vi "Find Relative Goal Location.vi"(10 "Goal Position":dbl[](array[numeric]), 11 "Current Position":dbl[](array[numeric])) -> (2 "Target Distance":dbl, 3 "Target Heading":dbl)   [LabVIEW 2017]
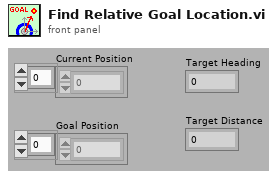
[diagram p1: front panel]
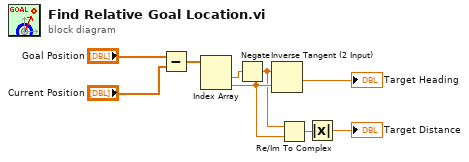
[diagram p0: block diagram]
diagram:
  n1 = Subtract(x="Goal Position", y="Current Position") -> (x-y=w9:dbl[])
  n2 = Index Array(array=w9) -> (element #1=w5:dbl, element #2=w6:dbl)  [unwired: 2 in]
  n3 = Negate(x=w5) -> (-x=w3:dbl)
  n4 = Inverse Tangent (2 Input)(1:w6, 2:w3) -> (0:→"Target Heading":dbl)
  n5 = Re/Im To Complex(1:w6, 2:w3) -> (0:w2:cdb)
  n6 = Absolute Value(x=w2) -> (abs(x)=→"Target Distance":dbl)
